vi "Write Multiple Coils.vi"(8 "error in (no error)":errorcluster, 9 "coil values":bool[](array[boolean]), 10 "starting address":u16, 11 "Modbus master in":refnum<class "Network Master.lvclass">) -> (0 "error out":errorcluster, 3 "Modbus master out":refnum<class "Network Master.lvclass">)   [LabVIEW 2021, in "Network Master.lvclass"]
doc: "Writes values to contiguous coils. The maximum number of coils this VI can write is 1,968."
uses:
  Network Master.lvclass
  Modbus Data Unit/Modbus Data Unit.lvclass/Modbus Data Unit.ctl
  Network Master.lvclass/Network Master.ctl
  Modbus Data Unit/Construct PDU.vi
  Utility/Bits to Bytes.vi
  Data Model/Error Generator.vi
  Master Function Definition/Function code mismatch error.vi
  Modbus Data Unit/Deconstruct PDU.vi
  Modbus Data Unit/Modbus Data Unit.lvclass
  Transmission Data Unit/Transmission Data Unit.lvclass
  Master Function Definition/Master Function Definition.lvclass
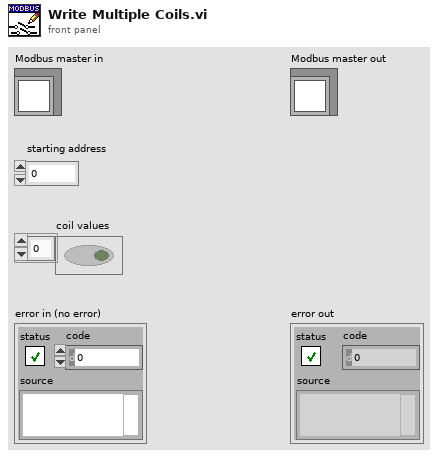
[diagram p1: front panel]
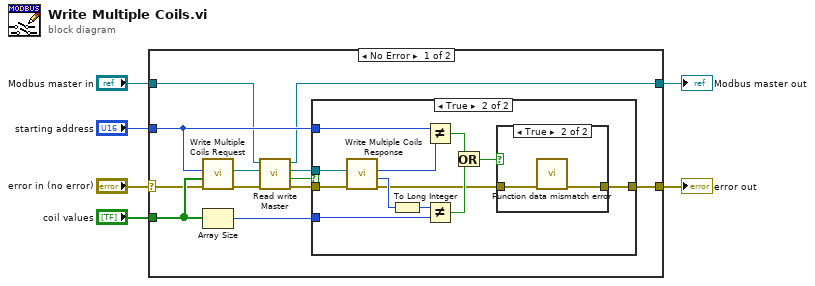
[diagram p0: block diagram]
diagram:
  n1 = case shown="No Error" "error in (no error)" {
    selector: "error in (no error)" -> [w7 w36]
    tunnel: "Modbus master in" -> [w8 w35]
    tunnel: [w17 w36] -> w5
    tunnel: [w9 w35] -> w6
    tunnel: "starting address" -> [w16 _]
    tunnel: "coil values" -> [w15 _]
    frame No Error {
      n2 = call "Write Multiple Coils Request.vi"("error in"=w7, "Coils To Write"=w15, "Starting Address"=w16) -> ("error out"=w18:errorcluster, "modbus data unit out"=w10:refnum<class "Modbus Data Unit.lvclass">)  [unwired: 7 in]
      n3 = Array Size(array=w15) -> (size(s)=w14:i32)
      n4 = call "Read write Master.vi"("error in (no error)"=w18, "Modbus data unit in"=w10, "Modbus master in"=w8) -> ("error out"=w13:errorcluster, "PDU valid?"=w12:bool, "Modbus data unit out"=w11:refnum<class "Modbus Data Unit.lvclass">, "Modbus master out"=w9:refnum<class "Network Master.lvclass">)  [unwired: 5 in]
      n5 = case shown="True" w12 {
        tunnel: [w19 w28] -> w17
        tunnel: w16 -> [_ w21]
        tunnel: w14 -> [_ w26]
        tunnel: w13 -> [w19 w25]
        tunnel: w11 -> [_ w24]
        frame False {
        }
        frame True {
          n6 = call "Write Multiple Coils Response.vi"("error in"=w25, "modbus data unit in"=w24) -> ("error out"=w23:errorcluster, "Number of Coils"=w27:u16, "Start Address"=w22:u16)  [unwired: 7 in]
          n7 = To Long Integer(number=w27) -> (32bit integer=w20:i32)
          n8 = Not Equal?(x=w21, y=w22) -> (x != y?=w30:bool)
          n9 = Not Equal?(x=w20, y=w26) -> (x != y?=w29:bool)
          n10 = Or(x=w30, y=w29) -> (x .or. y?=w31:bool)
          n11 = case shown="True" w31 {
            tunnel: [w32 w33] -> w28
            tunnel: w23 -> [w32 w34]
            frame False {
            }
            frame True {
              n12 = call "Function data mismatch error.vi"("error in (no error)"=w34) -> ("error out"=w33:errorcluster)  [unwired: 10 in]
            }
          }
        }
      }
    }
    frame Error {
    }
  }
  "error out" <- w5
  "Modbus master out" <- w6
